vi "TecellaRPCFormat.vi"(9 "Args":string[](array[string]), 10 "method":string, 11 "Name":string) -> (3 "The RPC string":string)   [LabVIEW 2009, in "TecellaClient.lvclass"]
uses:
  TecellaClient.lvclass
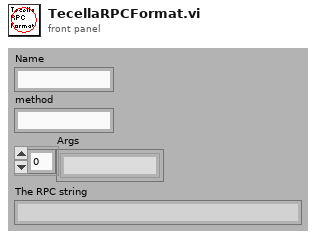
[diagram p1: front panel]
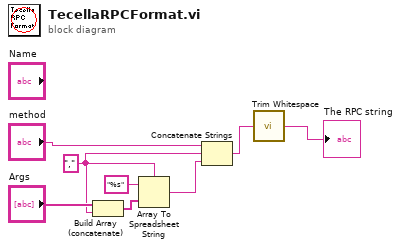
[diagram p0: block diagram]
diagram:
  w1 = "," ("delimiter (Tab)")
  n1 = Build Array (concatenate)("Args", w1) -> (w3:string[])
  n2 = Array To Spreadsheet String(delimiter (Tab)=w1, array=w3, 3:"%s" ("format string")) -> (spreadsheet string=w4:string)
  n3 = Concatenate Strings("method", w1, w4) -> (w6:string)
  n4 = call <vilib>:"Trim Whitespace.vi"("string"=w6) -> ("trimmed string"=→"The RPC string":string)  [unwired: 1 in]
